vi "Uninstall 1.0.vi"   [LabVIEW 2017, in "nisyscfg.lvlib"]
doc: "Uninstalls or installs software from a specified system."
uses:
  <vilib>/nisyscfg/nisyscfg.lvlib
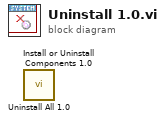
[diagram p0: block diagram]
diagram:
  n1 = call <vilib>:"Uninstall All 1.0.vi"() -> ()  [unwired: 10 in, 2 out]
  n2 = call <vilib>:"Install or Uninstall Components 1.0.vi"() -> ()  [unwired: 9 in, 3 out]
